vi "Max_forsed_bit64.vi"(3 "IN":u64 format="%b") -> (1 "N":u64 format="%b")   [LabVIEW 2019, in "Logik.lvlib"]
uses:
  Logik.lvlib
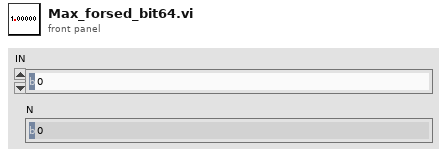
[diagram p1: front panel]
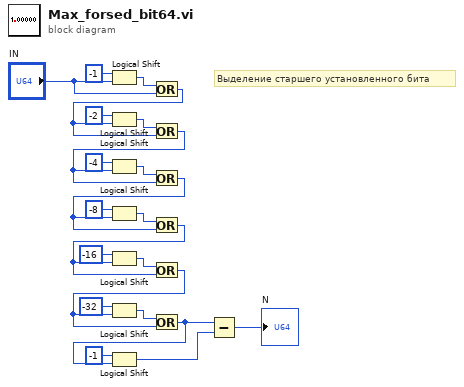
[diagram p0: block diagram]
diagram:
  # "Выделение старшего установленного бита"
  n1 = Logical Shift(y=i16 -1, x="IN") -> (x << y=w12:u64)
  n2 = Or(x=w12, y="IN") -> (x .or. y?=w11:u64)
  n3 = Logical Shift(y=i16 -2, x=w11) -> (x << y=w21:u64)
  n4 = Or(x=w21, y=w11) -> (x .or. y?=w10:u64)
  n5 = Logical Shift(y=i16 -4, x=w10) -> (x << y=w18:u64)
  n6 = Or(x=w18, y=w10) -> (x .or. y?=w9:u64)
  n7 = Logical Shift(y=i16 -8, x=w9) -> (x << y=w17:u64)
  n8 = Or(x=w17, y=w9) -> (x .or. y?=w3:u64)
  n9 = Logical Shift(y=i16 -16, x=w3) -> (x << y=w4:u64)
  n10 = Or(x=w4, y=w3) -> (x .or. y?=w2:u64)
  n11 = Logical Shift(y=i16 -32, x=w2) -> (x << y=w14:u64)
  n12 = Or(x=w14, y=w2) -> (x .or. y?=w8:u64)
  n13 = Logical Shift(y=i16 -1, x=w8) -> (x << y=w7:u64)
  n14 = Subtract(x=w8, y=w7) -> (x-y=→"N":u64)
